vi "AIT 1553 - Get Index and Length.vi"(11 "Section":T1 {"Message Settings"."Driver Data"."First Word" min=8 max=31; "Message Settings"."Driver Data"."Num Bits" min=1 max=32; "Message Settings"."Driver Data"."Start Bit" min=8 max=31; "Message Settings"."Block Data Refs"."Data Reference" format="%.0x"}) -> (2 "Length":i32, 3 "FIFO Index":i32)   [LabVIEW 2014, in "AIT 1553 Custom Device.lvlib"]
uses:
  AIT 1553 Custom Device.lvlib
  RT Controls/AIT 1553 - RT HW Channel.ctl
  RT Controls/AIT 1553 - Bus Section.ctl
  RT Controls/AIT 1553 - RT Message Settings.ctl
  <vilib>/NI Veristand/Custom Device API/Block Data Reference.ctl
  <vilib>/NI Veristand/Custom Device API/Data Reference.ctl
  RT Controls/AIT 1553 - Driver Data.ctl
  Controls and Global/Start Bit.ctl
  Controls and Global/Number of Bits.ctl
  <vilib>/NI Veristand/Custom Device API/Custom Device API.lvlib
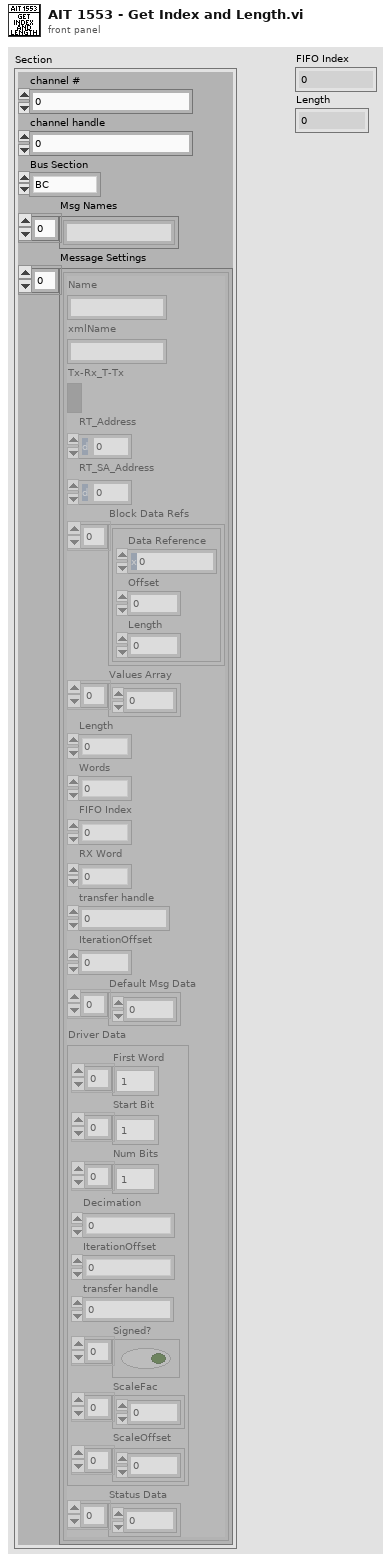
[diagram p1: front panel]
types:
  T1 = typedef "AIT 1553 Custom Device.lvlib/AIT 1553 - RT HW Channel.ctl" = cluster{"channel #":u16, "channel handle":u32, "Bus Section":T2, "Msg Names":string[], "Message Settings":T3[]}
  T2 = typedef "AIT 1553 Custom Device.lvlib/AIT 1553 - Bus Section.ctl" = enum16{"BC", "BM", "RT"}
  T3 = typedef "AIT 1553 Custom Device.lvlib/AIT 1553 - RT Message Settings.ctl" = cluster{"Name":string, "xmlName":string, "Tx-Rx_T-Tx":bool, "RT_Address":u8, "RT_SA_Address":u8, "Block Data Refs":T4[], "Values Array":dbl[], "Length":i32, "Words":i32, "FIFO Index":i32, "RX Word":u32, "transfer handle":u32, "IterationOffset":i32, "Default Msg Data":u16[], "Driver Data":T6, "Status Data":u32[]}
  T4 = typedef "Custom Device API.lvlib/Block Data Reference.ctl" = cluster{"Data Reference":T5, "Offset":i32, "Length":i32}
  T5 = typedef "Custom Device API.lvlib/Data Reference.ctl" = i32
  T6 = typedef "AIT 1553 Custom Device.lvlib/AIT 1553 - Driver Data.ctl" = cluster{"First Word":T7[], "Start Bit":T7[], "Num Bits":T8[], "Decimation":i32, "IterationOffset":i32, "transfer handle":u32, "Signed?":bool[], "ScaleFac":dbl[], "ScaleOffset":dbl[]}
  T7 = typedef "AIT 1553 Custom Device.lvlib/Start Bit.ctl" = i32
  T8 = typedef "AIT 1553 Custom Device.lvlib/Number of Bits.ctl" = i32
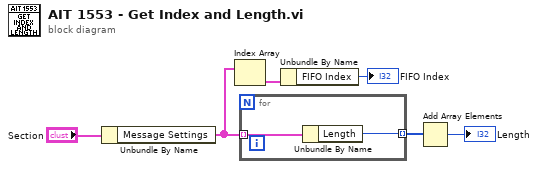
[diagram p0: block diagram]
diagram:
  n1 = Unbundle By Name("Section") -> ("Message Settings"=w4:T3[])
  n2 = Index Array(array=w4) -> (element=w5:T3)  [unwired: 1 in]
  n3 = for {
    tunnel: w4 -> [w8] mode=indexing
    tunnel: [w7] -> w6 mode=indexing
    n4 = Unbundle By Name(w8) -> ("Length"=w7:i32)
  }
  n5 = Unbundle By Name(w5) -> ("FIFO Index"=→"FIFO Index":i32)
  n6 = Add Array Elements(numeric array=w6) -> (sum=→"Length":i32)
